vi "Desktop Main.vi"() -> ()   [LabVIEW 2021]
doc: "Demonstrates the use of the Network Streams functions to send messages to the myRIO target."
uses:
  <vilib>/ErrorRing/Error Ring.xnode
  <resource>/objmgr/ni.dex.rc
panel:
  in  "Stop":bool
  in  "LED":bool[](array[boolean])=[FALSE, FALSE, FALSE, FALSE]
  out "error out":errorcluster
  in  "Target IP Address":string="172.22.11.2"
  # "Overview: Demonstrates the use of the Network Streams functions to send messages to the myRIO target.\nInstructions:\n1. Verify the value in Target IP Address. If it is incorrect, specify the correct value.\n2. Run this VI.\n3. Open RT Main.vi and follow its front panel instructions.\n4. Change the value of LED on this VI and observe the LEDs on the myRIO device and the value of LED Status on RT Main.vi. They change when the value of LED on this VI changes.\n5. Click Stop to stop this VI. Stopping this VI also terminates the running of RT Main.vi."
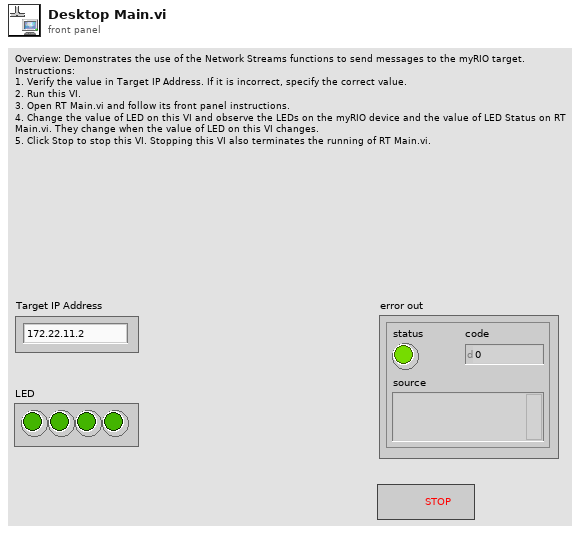
[diagram p1: front panel]
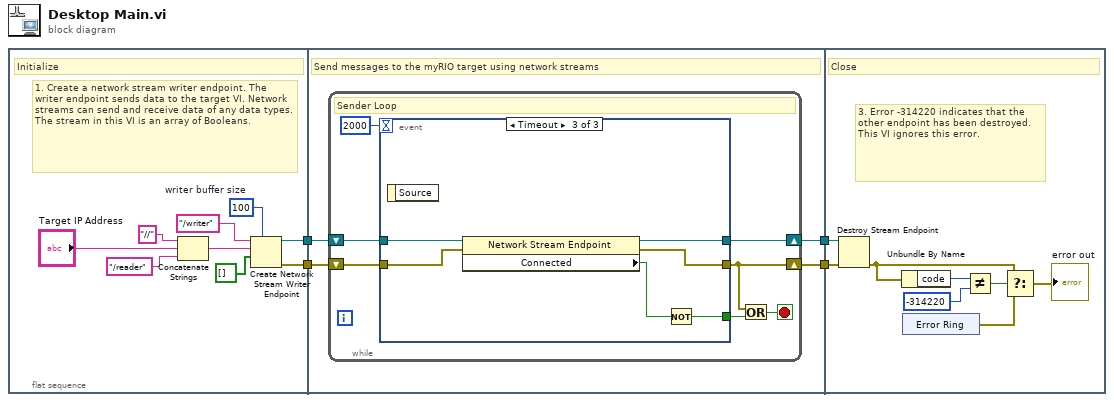
[diagram p0: block diagram]
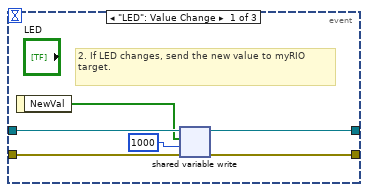
[diagram p2: hidden frame]
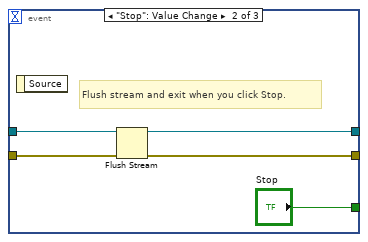
[diagram p3: hidden frame]
diagram:
  n1 = flat-sequence {
    tunnel: [w7] -> w4
    tunnel: [w6] -> w3
    tunnel: w4 -> [w17]
    tunnel: w3 -> [w16]
    tunnel: [w15] -> w2
    tunnel: [w14] -> w1
    tunnel: w2 -> [w43]
    tunnel: w1 -> [w42]
    frame #0 {
      w13 = 100  # writer buffer size
      # "1. Create a network stream writer endpoint. The writer endpoint sends data to the target VI. Network streams can send and receive data of any data types. The stream in this VI is an array of Booleans."
      # "Initialize"
      n2 = Concatenate Strings("//", "Target IP Address", "/reader") -> (w12:string)
      n3 = Create Network Stream Writer Endpoint(7:w13, 9:bool[] [], 10:w12, 11:"/writer" ("reader name")) -> (0:w6:errorcluster, 3:w7:refnum<k21>)  [unwired: 3 in]
    }
    frame #1 {
      # "Send messages to the myRIO target using network streams"
      n4 = while {
        shift-right: [w20] -> w14
        shift-left: w16 -> [w22]
        shift-right: [w23] -> w15
        shift-left: w17 -> [w24]
        stop <- w21 stop-if-true
        # "Sender Loop"
        n5 = event shown="[2] Timeout" {
          selector: _ -> [_ _ _]
          dyn-events: _ -> [_ _ _]
          timeout: 2000 -> [_ _ _]
          tunnel: w24 -> [w29 w34 w41]
          tunnel: [w30 w33 w40] -> w23
          tunnel: w22 -> [w28 w32 w39]
          tunnel: [w27 w31 w38] -> w20
          tunnel: [_ "Stop" w36] -> w19
          event "LED": Value Change {
            # "2. If LED changes, send the new value to myRIO target."
            n6 = event-data() -> ("NewVal"=w26:bool[])  [unwired: 1 in]
            n7 = shared-variable-write(w29, w28, w26, 1000 ("timeout ms (-1)")) -> (w30:refnum<k21>, w27:errorcluster)  [unwired: 1 out]
          }
          event "Stop": Value Change {
            # "Flush stream and exit when you click Stop."
            n8 = event-data() -> ()  [unwired: 1 in, 1 out]
            n9 = Flush Stream(8:w32, 11:w34) -> (0:w31:errorcluster, 3:w33:refnum<k21>)  [unwired: 2 in, 1 out]
          }
          event Timeout {
            n10 = event-data() -> ()  [unwired: 1 in, 1 out]
            n11 = property class="Network Stream Endpoint"(reference=w41, error in=w39) -> (reference out=w40:refnum<k21>, error out=w38:errorcluster, "Connected"=w37:bool)
            n12 = Not(x=w37) -> (.not. x?=w36:bool)
          }
        }
        n13 = Or(x=w20, y=w19) -> (x .or. y?=w21:bool)
      }
    }
    frame #2 {
      # "3. Error -314220 indicates that the other endpoint has been destroyed. This VI ignores this error."
      # "Close"
      n14 = Destroy Stream Endpoint(8:w42, 11:w43) -> (0:w49:errorcluster)
      n15 = Unbundle By Name(w49) -> ("code"=w48:i32)
      n16 = xnode "Error Ring"() -> ("error out"=w45:errorcluster)
      n17 = Not Equal?(x=w48, y=-314220) -> (x != y?=w46:bool)
      n18 = Select(t=w49, s=w46, f=w45) -> (s? t:f=→"error out":errorcluster)
    }
  }
